vi "Rohde & Schwarz VNA Get Stimulus.vi"(7 "Rohde & Schwarz VNA":T1, 8 "error in (no error)":errorcluster, 9 "Channel":i8=1, 11 "VISA Resource Name":refnum<visa-resource-name>) -> (0 "error out":errorcluster, 2 "SP Stimulus":T2={"Use Instrument Settings"=FALSE, "Blank Frequencies"=FALSE, "Sweep Type"=enum."Linear", "Sweep"={"Fstart"=500.0, "Fstop"=1500.0, "Units"=enum."MHz", "Points"=201}, "Power (dBm)"=999.0, "IFBW (Hz)"=-1.0, "Sweep Time (s)"=-1.0, "Calibration"={"State"=FALSE, "String"=""}} {"Sweep Time (s)" format="%.3g"}, 3 "dup VISA Resource Name":refnum<visa-resource-name>)   [LabVIEW 2011]
uses:
  tests/S Parameter/TypeDefs/SP Stimulus Parameters.ctl
  tests/S Parameter/TypeDefs/SP Frequency Units.ctl
  tests/S Parameter/TypeDefs/SP Calibration State.ctl
  TypeDefs/Rohde & Schwarz VNA Instrument Info.ctl
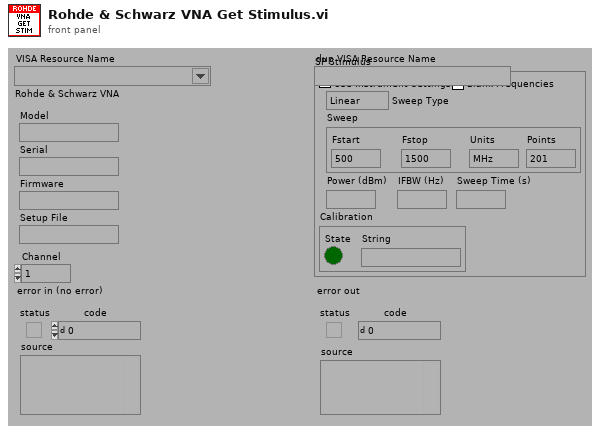
[diagram p1: front panel]
types:
  T1 = typedef "Rohde & Schwarz VNA Instrument Info.ctl" = cluster{"Model":string, "Serial":string, "Firmware":string, "Setup File":string}
  T2 = typedef "SP Stimulus Parameters.ctl" = cluster{"Use Instrument Settings":bool, "Blank Frequencies":bool, "Sweep Type":enum32{"Linear", "Logarithmic", "List", "Power", "CW"}, "Sweep":cluster{"Fstart":dbl, "Fstop":dbl, "Units":T3, "Points":i32}, "Power (dBm)":dbl, "IFBW (Hz)":dbl, "Sweep Time (s)":dbl, "Calibration":T4}
  T3 = typedef "SP Frequency Units.ctl" = enum16{"Hz", "kHz", "MHz", "GHz", "Points"}
  T4 = typedef "SP Calibration State.ctl" = cluster{"State":bool, "String":string}
  T5 = typedef "Rohde & Schwarz VNA Sweep Type.ctl" = enum32{"Linear", "Logarithmic", "Segmented", "Power", "Time", "CW"}
  T6 = enum32{"Linear", "Logarithmic", "List", "Power", "CW"}
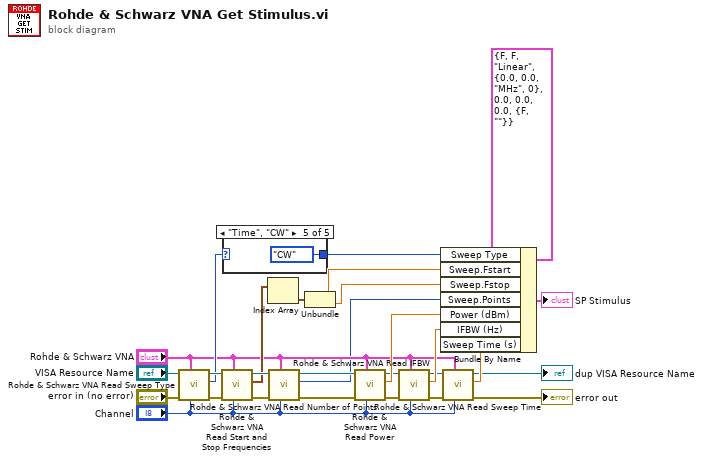
[diagram p0: block diagram]
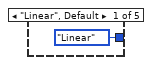
[diagram p2: hidden frame]
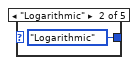
[diagram p3: hidden frame]
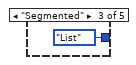
[diagram p4: hidden frame]
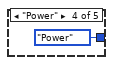
[diagram p5: hidden frame]
diagram:
  n1 = call "Rohde & Schwarz VNA Read Sweep Type.vi"("Channel"="Channel", "Rohde & Schwarz VNA"="Rohde & Schwarz VNA", "error in (no error)"="error in (no error)", "VISA Resource Name"="VISA Resource Name") -> ("error out"=w24:errorcluster, "Sweep Type"=w7:T5, "dup VISA Resource Name"=w23:refnum<visa-resource-name>)  [unwired: 5 out]
  n2 = call "Rohde & Schwarz VNA Read Start and Stop Frequencies.vi"("Channel"="Channel", "Rohde & Schwarz VNA"="Rohde & Schwarz VNA", "error in (no error)"=w24, "VISA Resource Name"=w23) -> ("error out"=w21:errorcluster, "Start/Stop Freqs, MHz"=w19:cluster{"Fstart":dbl, "Fstop":dbl}[], "dup VISA Resource Name"=w20:refnum<visa-resource-name>)  [unwired: 5 out]
  n3 = case shown="\"Time\", \"CW\"" w7 {
    tunnel: [T6."Linear" ("Sweep Type") T6."Logarithmic" ("Sweep Type") T6."List" ("Sweep Type") T6."Power" ("Sweep Type") T6."CW" ("Sweep Type")] -> w1
    frame "Linear", Default {
    }
    frame "Logarithmic" {
    }
    frame "Segmented" {
    }
    frame "Power" {
    }
    frame "Time", "CW" {
    }
  }
  n4 = Index Array(array=w19) -> (element=w8:cluster{"Fstart":dbl, "Fstop":dbl})  [unwired: 1 in]
  n5 = call "Rohde & Schwarz VNA Read Number of Points.vi"("Channel"="Channel", "Rohde & Schwarz VNA"="Rohde & Schwarz VNA", "error in (no error)"=w21, "VISA Resource Name"=w20) -> ("error out"=w15:errorcluster, "Number Points"=w2:i32, "dup VISA Resource Name"=w16:refnum<visa-resource-name>)  [unwired: 5 out]
  n6 = Unbundle(w8) -> ("Fstart"=w4:dbl, "Fstop"=w3:dbl)
  n7 = call "Rohde & Schwarz VNA Read Power.vi"("Channel"="Channel", "Rohde & Schwarz VNA"="Rohde & Schwarz VNA", "error in (no error)"=w15, "VISA Resource Name"=w16) -> ("error out"=w17:errorcluster, "Source Power, dBm"=w26:dbl, "dup VISA Resource Name"=w18:refnum<visa-resource-name>)  [unwired: 5 out]
  n8 = call "Rohde & Schwarz VNA Read IFBW.vi"("Channel"="Channel", "Rohde & Schwarz VNA"="Rohde & Schwarz VNA", "error in (no error)"=w17, "VISA Resource Name"=w18) -> ("error out"=w13:errorcluster, "IFBW, Hz"=w27:dbl, "dup VISA Resource Name"=w14:refnum<visa-resource-name>)  [unwired: 5 out]
  n9 = call "Rohde & Schwarz VNA Read Sweep Time.vi"("Channel"="Channel", "Rohde & Schwarz VNA"="Rohde & Schwarz VNA", "error in (no error)"=w13, "VISA Resource Name"=w14) -> ("error out"=→"error out":errorcluster, "Sweep Time, s"=w12:dbl, "dup VISA Resource Name"=→"dup VISA Resource Name":refnum<visa-resource-name>)  [unwired: 5 out]
  n10 = Bundle By Name(cluster=T2 {"Use Instrument Settings"=FALSE, "Blank Frequencies"=FALSE, "Sweep Type"=enum."Linear", "Sweep"={"Fstart"=0.0, "Fstop"=0.0, "Units"=enum."MHz", "Points"=0}, "Power (dBm)"=0.0, "IFBW (Hz)"=0.0, "Sweep Time (s)"=0.0, "Calibration"={"State"=FALSE, "String"=""}} ("Stimulus"), "Sweep Type"=w1, "Sweep.Fstart"=w4, "Sweep.Fstop"=w3, "Sweep.Points"=w2, "Power (dBm)"=w26, "IFBW (Hz)"=w27, "Sweep Time (s)"=w12) -> (→"SP Stimulus":T2)
